vi "Read Image.vi"(8 "error in (no error)":errorcluster, 11 "New Image Msg in":refnum<class "New Image Msg.lvclass">) -> (0 "error out":errorcluster, 1 "Buffer Number":u32, 2 "Image":T1, 3 "New Image Msg out":refnum<class "New Image Msg.lvclass">)   [LabVIEW 2014, in "Camera Actor.lvlib" / "New Image Msg.lvclass"]
uses:
  New Image Msg.lvclass
  <vilib>/vision/Image Controls.llb/IMAQ Image.ctl
  New Image Msg.lvclass/New Image Msg.ctl
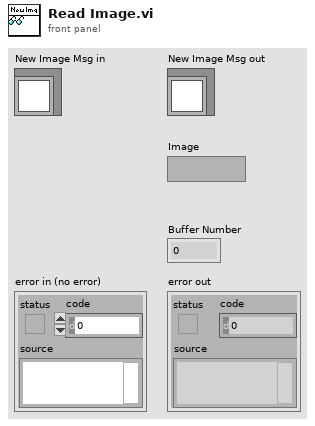
[diagram p1: front panel]
types:
  T1 = typedef "IMAQ Image.ctl" = refnum<image>
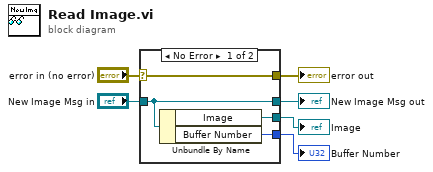
[diagram p0: block diagram]
diagram:
  n1 = case shown="No Error" "error in (no error)" {
    selector: "error in (no error)" -> [w10 w11]
    tunnel: [w10 w11] -> w5
    tunnel: [w9 w12] -> w3
    tunnel: "New Image Msg in" -> [w9 w12]
    tunnel: [w8 _] -> w2
    tunnel: [w7 _] -> w1
    frame No Error {
      n2 = Unbundle By Name(w9) -> ("Image"=w8:T1, "Buffer Number"=w7:u32)
    }
    frame Error {
    }
  }
  "error out" <- w5
  "New Image Msg out" <- w3
  "Image" <- w2
  "Buffer Number" <- w1
